vi "Add NI-XNET CAN Hardware_Add Signal.vi"(8 "error in (no error)":errorcluster, 10 "Signals":T1[](array[typedef]), 11 "Frame Ref":refnum<k24>) -> (0 "error out":errorcluster, 3 "Frame Ref out":refnum<k24>)   [LabVIEW 2019, in "Simple SysDef API.lvlib"]
uses:
  <userlib>/SimpleSysDef/Simple SysDef API.lvlib
  <userlib>/SimpleSysDef/_SubVIs/Add NI-XNET CAN Hardware_Signal Settings.ctl
  NationalInstruments.VeriStand.SystemDefinitionAPI
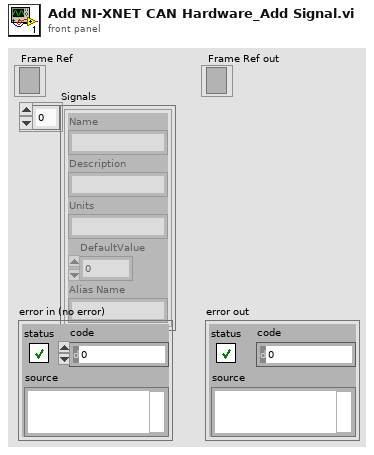
[diagram p1: front panel]
types:
  T1 = typedef "Simple SysDef API.lvlib/Add NI-XNET CAN Hardware_Signal Settings.ctl" = cluster{"Name":string, "Description":string, "Units":string, "DefaultValue":dbl, "Alias Name":string}
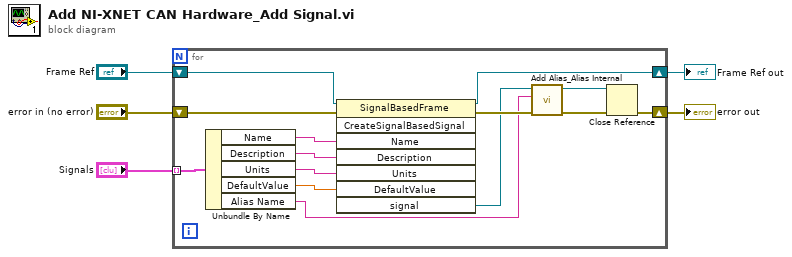
[diagram p0: block diagram]
diagram:
  n1 = for {
    shift-right: [w16] -> w4
    shift-left: "error in (no error)" -> [w18]
    shift-right: [w17] -> w3
    shift-left: "Frame Ref" -> [w19]
    tunnel: "Signals" -> [w15] mode=indexing
    n2 = Unbundle By Name(w15) -> ("Name"=w14:string, "Description"=w13:string, "Units"=w12:string, "DefaultValue"=w11:dbl, "Alias Name"=w6:string)
    n3 = invoke class="SignalBasedFrame" method="CreateSignalBasedSignal"(reference=w19, error in=w18, "Name"=w14, "Description"=w13, "Units"=w12, "DefaultValue"=w11) -> (reference out=w17:refnum<k24>, error out=w10:errorcluster, "signal"=w8:refnum<k24>)  [unwired: 2 in, 5 out]
    n4 = call <userlib>:"Add Alias_Alias Internal.vi"("error in (no error)"=w10, "Name"=w6, "Base Node"=w8) -> ("error out"=w9:errorcluster, "Base Node out"=w7:refnum<k24>)  [unwired: 7 in]
    n5 = Close Reference(reference=w7, error in (no error)=w9) -> (error out=w16:errorcluster)
  }
  "error out" <- w4
  "Frame Ref out" <- w3
